vi "MouseChirp-FM Sweep comparison.vi"() -> ()   [LabVIEW 2015]
uses:
  Controls/Level XCtl/Level Modes.ctl
  Controls/Level XCtl/Level Data.ctl
  Controls/Level XCtl/Level XCtl.xctl
  Controls/Level XCtl/Level Units.ctl
  Waveform VIs/FM Sweep VIs/FM Sweep Params.ctl
panel:
  out "Max SPL":dbl
  out "Max Level":dbl
  in  "FMSweep In":T1={"Rate (oct/s)"=42900000.0, "Fmin (Hz)"=100.0, "Fmax (Hz)"=60000.0, "Ramp (ms)"=0.1, "Linear"=TRUE}
  out "Waveform Graph":cluster{i32, "dx":dbl, "Array":dbl[]}[](graph)
  in  "Fs (Hz)":dbl=200000.0
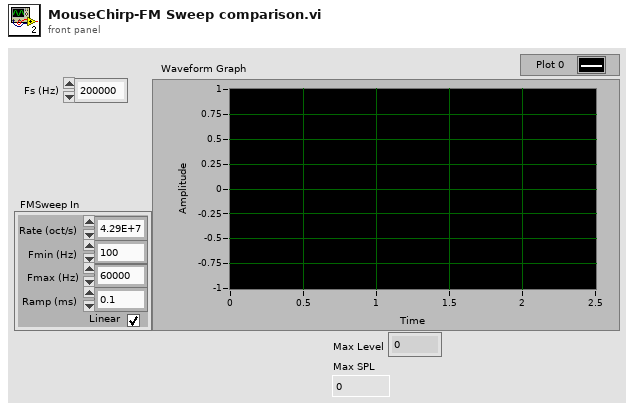
[diagram p1: front panel]
types:
  T1 = typedef "FM Sweep Params.ctl" = cluster{"Rate (oct/s)":dbl, "Fmin (Hz)":dbl, "Fmax (Hz)":dbl, "Ramp (ms)":dbl, "Linear":bool}
  T2 = typedef "Level Modes.ctl" = enum16{"dB atten", "dB SPL", "dB re 1 Vrms", "dB V/Hz½"}
  T3 = typedef "Level XCtl.xctl/Level Data.ctl" = cluster{"Level":dbl, "Units":T4, "Max":dbl, "Multiplier":dbl, "Cal File":path, "Cal":cluster{"Freq (Hz)":dbl[], "Mag (dB SPL)":dbl[], "Phase (deg)":dbl[]}}
  T4 = typedef "Level Units.ctl" = enum16{"dB atten", "dB SPL", "dB re 1 Vrms", "dB V/Hz½", "mW", "dB SL"}
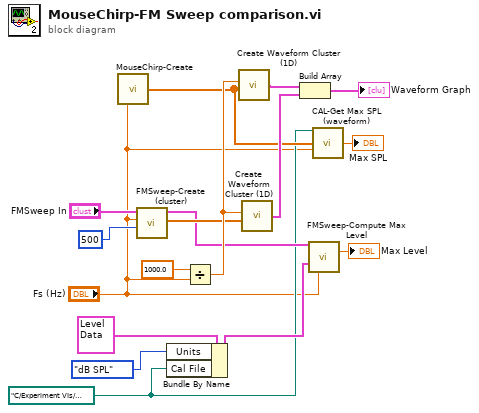
[diagram p0: block diagram]
diagram:
  w3 = path "C:/Experiment VIs/Signal Synthesis VIs/Test VIs/LeftPrimary_Eq_06Mar14.calib" ("Cal File")
  n1 = call "MouseChirp-Create.vi"("Fs (Hz)"="Fs (Hz)") -> ("Array"=w4:dbl[])  [unwired: 13 in, 1 out]
  n2 = call "FMSweep-Create (cluster).vi"("Npts"=500, "Sampling Rate (Hz)"="Fs (Hz)", "FMSweep In"="FMSweep In") -> ("Waveform"=w12:dbl[], "FMSweep Out"=w9:T1)  [unwired: 6 in, 1 out]
  n3 = Bundle By Name(cluster=T3 {"Level"=0.0, "Units"=enum."dB atten", "Max"=0.0, "Multiplier"=0.0, "Cal File"=path "", "Cal"={"Freq (Hz)"=[], "Mag (dB SPL)"=[], "Phase (deg)"=[]}} ("Level"), "Units"=Level_Modes."dB SPL" ("Mode"), "Cal File"=w3) -> (w7:T3)
  n4 = Divide(x=1000.0, y="Fs (Hz)") -> (x/y=w13:dbl)
  n5 = call "Create Waveform Cluster (1D).vi"("Array"=w4, "dx"=w13) -> ("waveform cluster"=w16:cluster{i32, "dx":dbl, "Array":dbl[]})  [unwired: 2 in]
  n6 = call "Create Waveform Cluster (1D).vi"("Array"=w12, "dx"=w13) -> ("waveform cluster"=w10:cluster{i32, "dx":dbl, "Array":dbl[]})  [unwired: 2 in]
  n7 = Build Array(w16, w10) -> (→"Waveform Graph":cluster{i32, "dx":dbl, "Array":dbl[]}[])
  n8 = call "FMSweep-Compute Max Level.vi"("FMSweep"=w9, "Level"=w7, "Fs (Hz)"="Fs (Hz)") -> ("Max Level"=→"Max Level":dbl)  [unwired: 10 in, 2 out]
  n9 = call "CAL-Get Max SPL (waveform).vi"("Cal File"=w3, "Y"=w4, "Sampling Rate (Hz)"="Fs (Hz)") -> ("Max SPL"=→"Max SPL":dbl)  [unwired: 11 in, 1 out]
